vi "Popup - Test Info.vi"(8 "error i":errorcluster) -> (0 "error out":errorcluster, 3 "Test Information out":T1={"APU Part Number:"="", "Model:"="", "Serial Number:"="", "Customer:"="", "Work Order:"="", "Pre or Post SB"="", "Run Count"=0, "APU Selected"="<Select>"} {"Run Count" min=0 step=1})   [LabVIEW 2018, in "Controller (Host).lvlib"]
doc: "This is the dialog used by the user to select an APU to test."
uses:
  Controller (Host).lvlib
  Public Controls/Test Information.ctl
  Public VIs/PreorPostSB.ctl
  Public Controls/APU Select.ctl
panel:
  in  "Test Information":T1={"APU Part Number:"="", "Model:"="", "Serial Number:"="", "Customer:"="", "Work Order:"="", "Pre or Post SB"="Post SB 49-7711", "Run Count"=0, "APU Selected"="<Select>"} {"Run Count" min=0 step=1}
  in  "Done":bool
  # "Test Information"
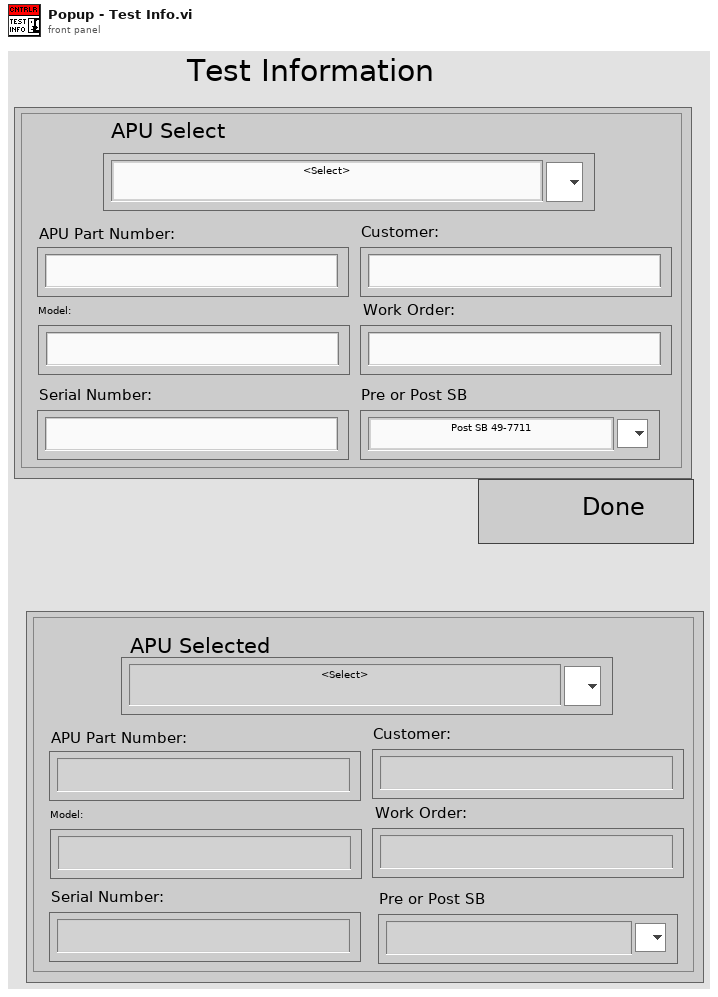
[diagram p1: front panel]
types:
  T1 = typedef "Controller (Host).lvlib/Test Information.ctl" = cluster{"APU Part Number:":string, "Model:":string, "Serial Number:":string, "Customer:":string, "Work Order:":string, "Pre or Post SB":T2, "Run Count":i32, "APU Selected":T3}
  T2 = typedef "Controller (Host).lvlib/PreorPostSB.ctl" = string
  T3 = typedef "Controller (Host).lvlib/APU Select.ctl" = string
  T4 = enum8{"Enabled", "Disabled", "Disabled and Grayed Out"}
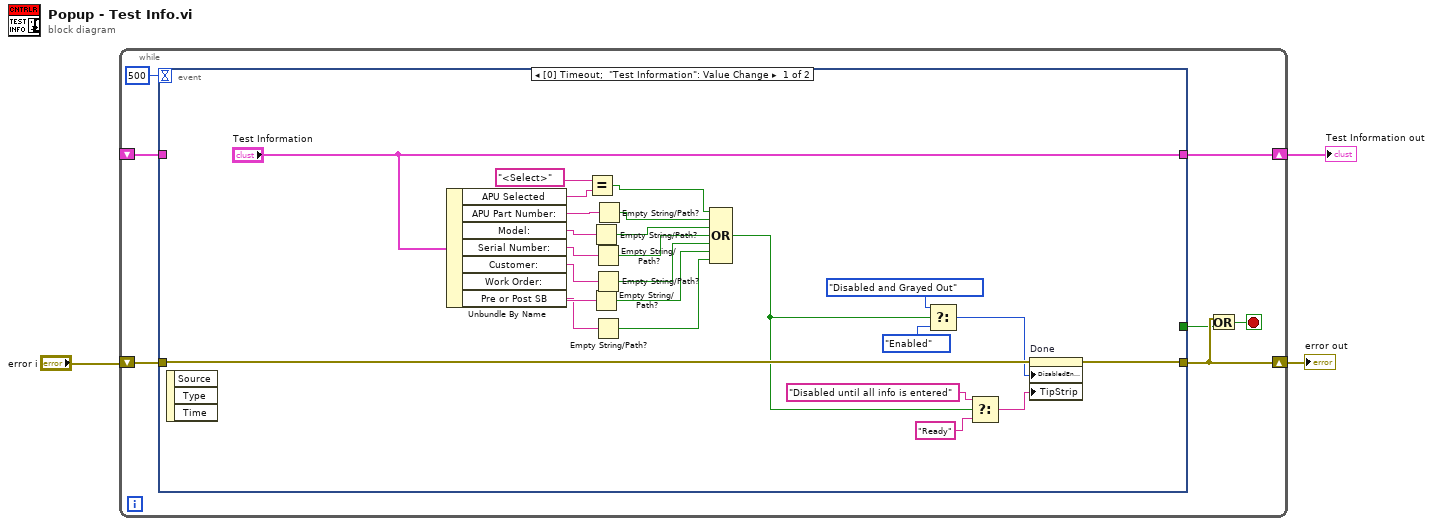
[diagram p0: block diagram]
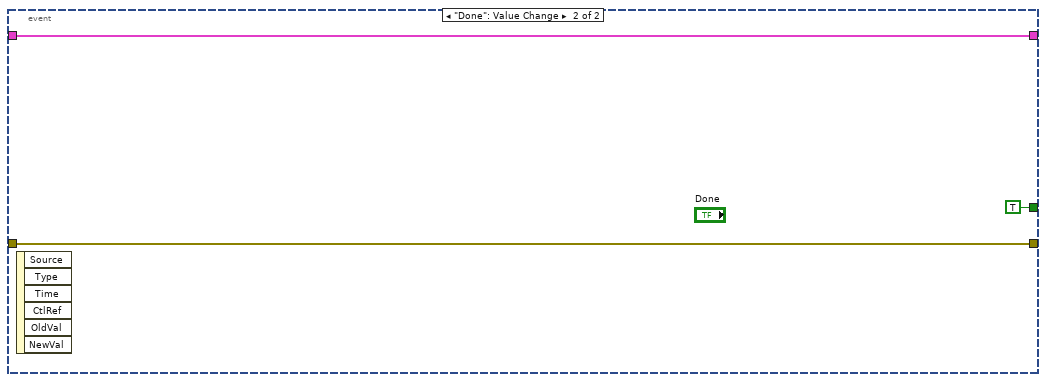
[diagram p2: hidden frame]
diagram:
  n1 = while {
    shift-right: [w9] -> w3
    shift-left: "error i" -> [w10]
    shift-right: [w6] -> w1
    shift-left: _ -> [w4]
    stop <- w7 stop-if-true
    n2 = event shown="[0] Timeout;  \"Test Information\": Value Change" {
      selector: _ -> [_ _]
      dyn-events: _ -> [_ _]
      timeout: 500 -> [_ _]
      tunnel: w10 -> [w23 w38]
      tunnel: [_ TRUE] -> w8
      tunnel: [w19 w38] -> w9
      tunnel: ["Test Information" w36] -> w6
      tunnel: w4 -> [_ w36]
      event Timeout; Value Change {
        n3 = event-data() -> ()  [unwired: 1 in, 3 out]
        n4 = Unbundle By Name("Test Information") -> ("APU Selected"=w13:T3, "APU Part Number:"=w35:string, "Model:"=w34:string, "Serial Number:"=w33:string, "Customer:"=w32:string, "Work Order:"=w31:string, "Pre or Post SB"=w25:T2)
        n5 = Equal?(x=T3 "<Select>" ("APU Select"), y=w13) -> (x = y?=w11:bool)
        n6 = Empty String/Path?(string/path=w34) -> (empty?=w29:bool)
        n7 = Empty String/Path?(string/path=w31) -> (empty?=w26:bool)
        n8 = Empty String/Path?(string/path=w33) -> (empty?=w28:bool)
        n9 = Empty String/Path?(string/path=w32) -> (empty?=w27:bool)
        n10 = Empty String/Path?(string/path=w25) -> (empty?=w24:bool)
        n11 = Empty String/Path?(string/path=w35) -> (empty?=w30:bool)
        n12 = Compound Arithmetic op=OR(w11, w30, w29, w28, w27, w26, w24) -> (w18:bool)
        n13 = Select(t=T4."Disabled and Grayed Out" ("Disabled"), s=w18, f=T4."Enabled" ("Disabled")) -> (s? t:f=w20:T4)
        n14 = Select(t="Disabled until all info is entered" ("Tip Strip"), s=w18, f="Ready" ("Tip Strip")) -> (s? t:f=w15:string)
        n15 = property on="Done" class="Bool"(error in=w23, "DisabledEnum"=w20, "TipStrip"=w15) -> (error out=w19:errorcluster)  [unwired: 1 in, 1 out]
      }
      event "Done": Value Change {
        n16 = event-data() -> ()  [unwired: 1 in, 6 out]
      }
    }
    n17 = Or(x=w9, y=w8) -> (x .or. y?=w7:bool)
  }
  "error out" <- w3
  "Test Information out" <- w1
